vi "Ballard XML Generator.Open Rx Channel.vi"(7 "other params":string[](array[string]), 10 "speedKHz":i32, 11 "string in":string) -> (3 "string out":string)   [LabVIEW 2017]
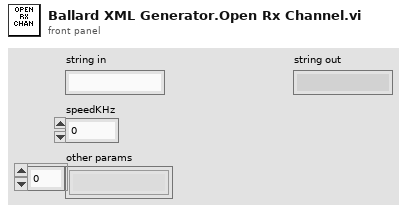
[diagram p1: front panel]
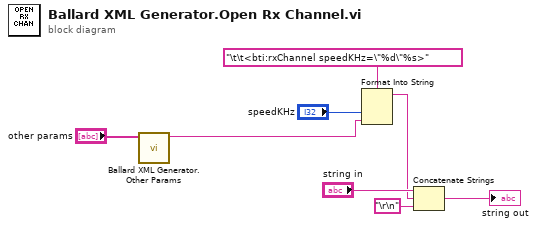
[diagram p0: block diagram]
diagram:
  n1 = call "Ballard XML Generator.Other Params.vi"("other params"="other params") -> ("string"=w1:string)  [unwired: 10 in]
  n2 = Format Into String(format string="\t\t<bti:rxChannel speedKHz=\"%d\"%s>", "speedKHz", w1) -> (resulting string=w4:string)  [unwired: 2 in, 1 out]
  n3 = Concatenate Strings("string in", w4, "\r\n") -> (→"string out":string)
